vi "LIDAR V3 Mem2 Manager.vi"(11 "Source Name":refnum<k21>="100 MHz Clock") -> ()   [LabVIEW 2013]
uses:
  <vilib>/Platform/TimedLoop/XDataNode/wakeup.ctl
  <vilib>/Platform/TimedLoop/XDataNode/XDNodeRunTimeDep.lvlib
  <vilib>/Platform/TimedLoop/XDataNode/nitl_modes.ctl
  <vilib>/Platform/TimedLoop/XDataNode/timing_clust.ctl
  <vilib>/Platform/TimedLoop/XDataNode/XDataNode.xnode
  <vilib>/rvi/DataTransferAndStorage/Container/XNode/niFpgaContainer.xnode
  <vilib>/rvi/FXPMathLib/FxpAdd/XNode/nifxpmath_Add.xnode
  <vilib>/rvi/FXPMathLib/sim/FxpSim.dll
  <vilib>/rvi/LocalResourceManager/LocalResourceManager.xnode
  <vilib>/rvi/FIFO/Fifo_Resource/niFpgaFifoEmulationRefIn.vi
  <vilib>/rvi/FIFO/Fifo_Resource/nirvififoEmulationRead.vi
  <vilib>/rvi/FIFO/Fifo_Resource/nirvififoEmulationWrite.vi
  <vilib>/rvi/Memory/Memory_Emulation/nirvimemoryFastEmulation.vi
  <vilib>/rvi/Memory/Memory_Emulation/nirvimemoryEmulation.vi
  <vilib>/rvi/DataTransferAndStorage/Container/Common/niFpgaContainerGetUniqueNameForEmu.vi
  <vilib>/rvi/DataTransferAndStorage/Container/Common/niFpgaContainerSetEmuInfo.vi
  <vilib>/rvi/eio/common/nirviEmuReportErrorAndStop.vi
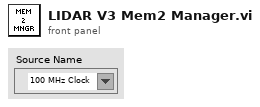
[diagram p1: front panel]
types:
  T1 = typedef "XDNodeRunTimeDep.lvlib/timing_clust.ctl" = cluster{"Expected End [f-1]":u64, "Actual End [f-1]":u64, "Finished Late? [f-1]":bool, "Expected End [i-1]":u64, "Actual End [i-1]":u64, "Finished Late? [i-1]":bool, "Expected Start [i]":u64, "Actual Start [i]":u64, "Expected Start [f]":u64, "Actual Start [f]":u64, "Source Name":string, "Structure Name":string, "Period":i64, "Deadline":i64, "Offset":i64, "Start":i64, "Priority":i32, "Timeout":i32, "Mode":T2, "Wakeup Reason":T3, "Error":errorcluster, "Source Type":string, "Secondary Source Type":string, "Global End Time":u64, "Global Start Time":u64, "Frame Duration":u64, "Iteration Duration":u64, "Assigned CPU":i32, "I/O Scan Engine Mode":u32}
  T2 = typedef "XDNodeRunTimeDep.lvlib/nitl_modes.ctl" = enum32{"No Change", "Process missed periods, maintain original phase", "Discard missed periods, maintain original phase", "Process missed periods, ignore original phase", "Discard missed periods, ignore original phase"}
  T3 = typedef "XDNodeRunTimeDep.lvlib/wakeup.ctl" = enum32{"Normal", "Aborted", "Asynchronous wakeup", "Timing source error", "Timed loop error", "Timeout"}
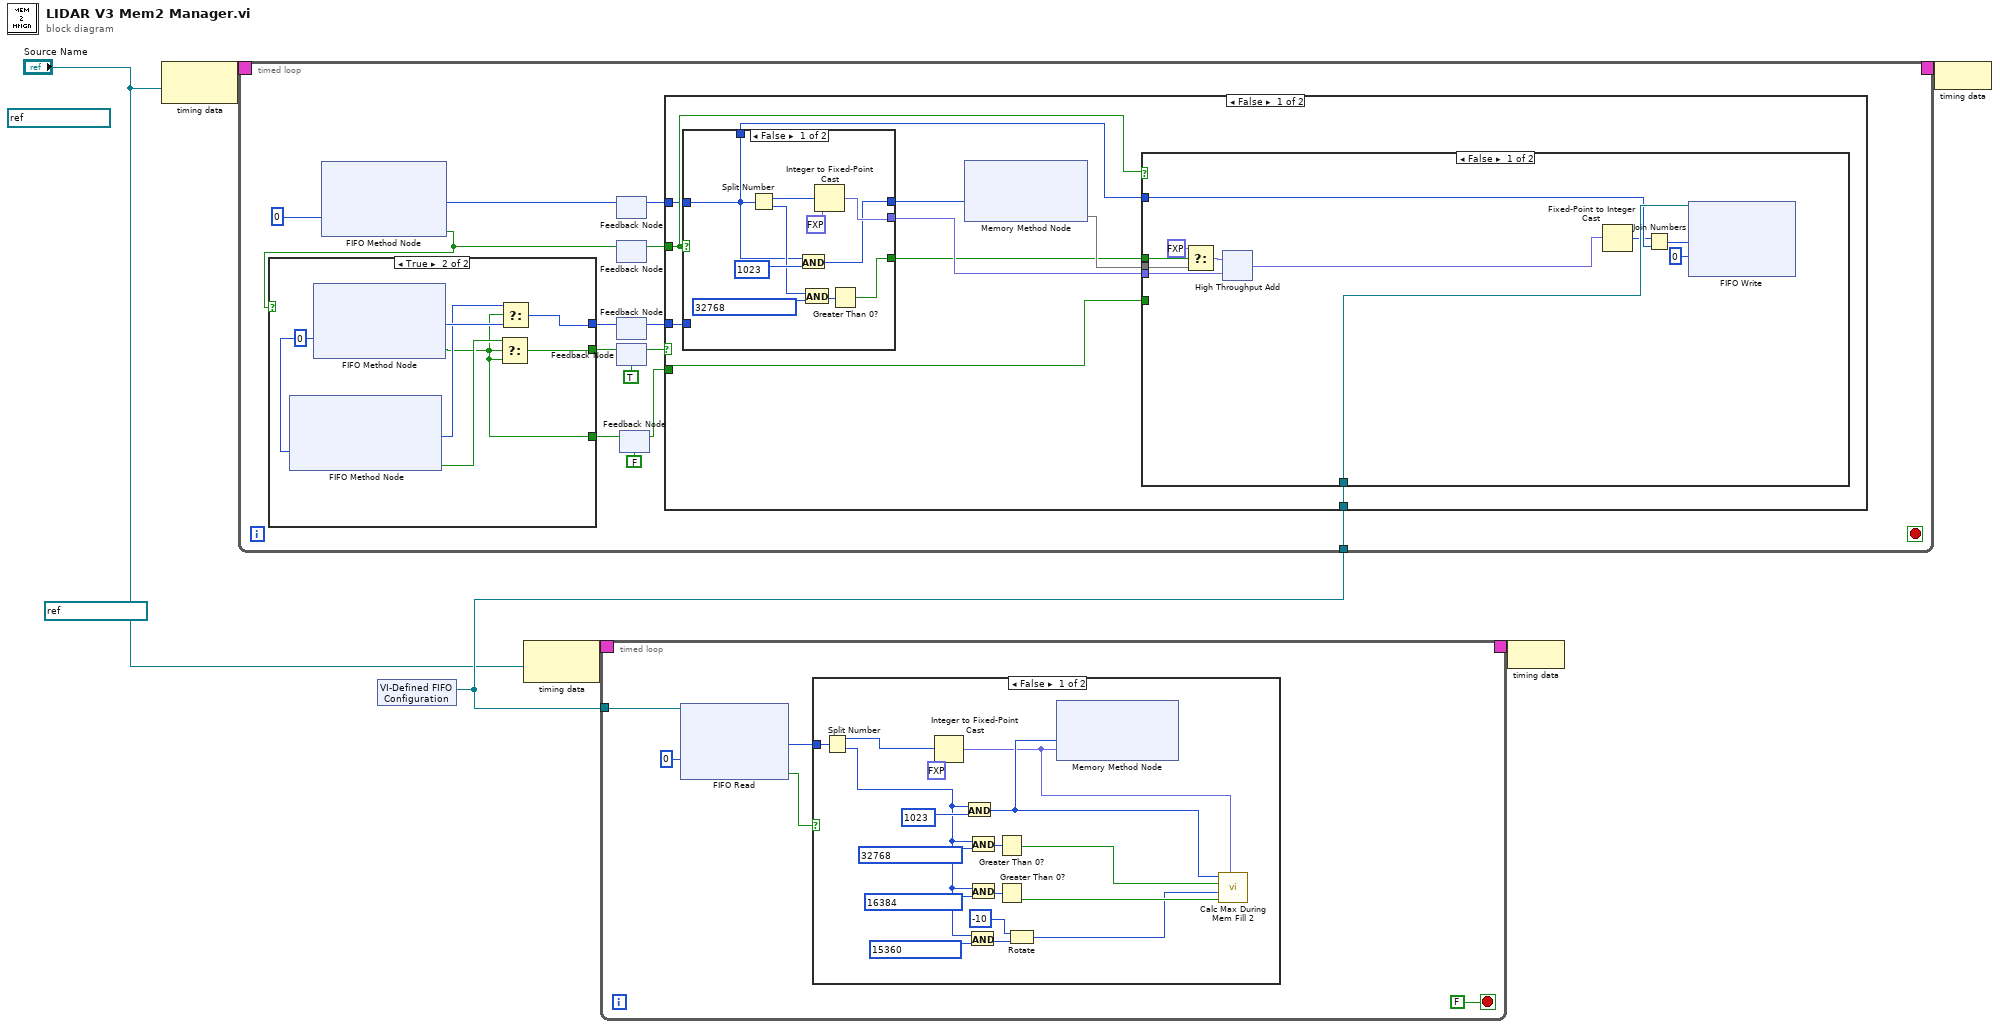
[diagram p0: block diagram]
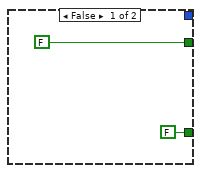
[diagram p3: hidden frame]
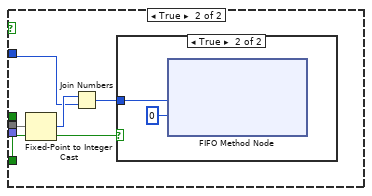
[diagram p4: hidden frame]
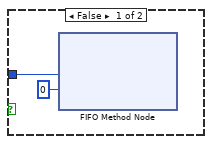
[diagram p5: hidden frame]
diagram:
  (unwired) refnum<k21> "100 MHz Clock" ("Source Name")
  (unwired) refnum<k21> "100 MHz Clock" ("Source Name")
  n1 = node-c288("Source Name") -> (w6:T1)
  n2 = xnode "VI-Defined FIFO Configuration"() -> ("FIFO Out"=w4:refnum<k21>)
  n3 = timed-loop {
    timing: w6 -> [_]
    timing-out: [_] -> w5
    tunnel: w4 -> [w15]
    stop <- _ stop-if-true
    n4 = xnode ("FIFO Method Node")("Timeout"=0) -> ("Element"=w20:u32, "Timed Out?"=w17:bool)  [unwired: 1 in, 1 out]
    n5 = case shown="True" w17 {
      tunnel: [FALSE ("Timed Out?") w28] -> w18
      tunnel: [_ w24] -> w16
      tunnel: [FALSE ("Timed Out?") w23] -> w9
      frame False {
      }
      frame True {
        w26 = 0 ("Timeout")
        n6 = xnode ("FIFO Method Node")("Timeout"=w26) -> ("Element"=w25:u32, "Timed Out?"=w29:bool)  [unwired: 1 in, 1 out]
        n7 = xnode ("FIFO Method Node")("Timeout"=w26) -> ("Element"=w27:u32, "Timed Out?"=w23:bool)  [unwired: 1 in, 1 out]
        n8 = Select(t=w29, s=w23, f=w23) -> (s? t:f=w28:bool)
        n9 = Select(t=w25, s=w23, f=w27) -> (s? t:f=w24:u32)
      }
    }
    n10 = feedback-in #1(w20) -> ()
    n11 = feedback #1() -> (w14:u32)  [unwired: 1 in]
    n12 = feedback-in #2(w17) -> ()
    n13 = feedback #2() -> (w13:bool)  [unwired: 1 in]
    n14 = feedback-in #3(w16) -> ()
    n15 = feedback #3() -> (w12:u32)  [unwired: 1 in]
    n16 = feedback-in #4(w18) -> ()
    n17 = feedback #4(TRUE ("Timed Out?")) -> (w11:bool)
    n18 = feedback #5(FALSE ("Timed Out?")) -> (w8:bool)
    n19 = feedback-in #5(w9) -> ()
    n20 = case shown="False" w11 {
      tunnel: w14 -> [w32 _]
      tunnel: w13 -> [w36 _]
      tunnel: w12 -> [w37 _]
      tunnel: w15 -> [w33 _]
      tunnel: w8 -> [w31 _]
      frame False {
        n21 = case shown="False" w36 {
          tunnel: w32 -> [w60 _]
          tunnel: [w69 _] -> w38
          tunnel: [w67 w70] -> w34
          tunnel: w37 -> [_ w70]
          tunnel: [w63 _] -> w35
          tunnel: [w60 w70] -> w30
          frame False {
            n22 = Split Number(x=w60) -> (hi(x)=w62:u16, lo(x)=w61:u16)
            n23 = And(x=w60, y=u32 1023) -> (x .and. y?=w67:u32)
            n24 = And(x=w61, y=u16 32768) -> (x .and. y?=w64:u16)
            n25 = Integer to Fixed-Point Cast(fixed-point type=fxp<+/-,16,16> 0.0, integer=w62) -> (fixed-point=w69:fxp<+/-,16,16>)
            n26 = Greater Than 0?(x=w64) -> (x > 0?=w63:bool)
          }
          frame True {
          }
        }
        n27 = xnode ("Memory Method Node")("Address"=w34) -> ("Data"=w39)  [unwired: 1 in, 1 out]
        n28 = case shown="False" w36 {
          tunnel: w39 -> [w48 w55]
          tunnel: w38 -> [w50 _]
          tunnel: w30 -> [w43 w52]
          tunnel: w35 -> [w44 _]
          tunnel: w33 -> [w45 _]
          tunnel: w31 -> [_ w51]
          frame False {
            n29 = Select(t=fxp<+/-,22,22> 0.0, s=w44, f=w48) -> (s? t:f=w47:fxp<+/-,22,22>)
            n30 = xnode ("High Throughput Add")("x"=w47, "y"=w50) -> ("x+y"=w46:fxp<+/-,22,22>)
            n31 = Fixed-Point to Integer Cast(1:w46) -> (0:w40:i32)
            n32 = Join Numbers(hi=w40, lo=w43) -> ((hi.lo)=w41:u64)
            n33 = xnode ("FIFO Write")("Element"=w41, "Timeout"=0, "FIFO In"=w45) -> ()  [unwired: 2 out]
          }
          frame True {
            n34 = Fixed-Point to Integer Cast(1:w55) -> (0:w53:i32)
            n35 = Join Numbers(hi=w53, lo=w52) -> ((hi.lo)=w54:u64)
            n36 = case shown="True" w51 {
              tunnel: w54 -> [w56 w58]
              frame False {
                n37 = xnode ("FIFO Method Node")("Element"=w56, "Timeout"=0) -> ()  [unwired: 1 in, 2 out]
              }
              frame True {
                n38 = xnode ("FIFO Method Node")("Element"=w58, "Timeout"=0) -> ()  [unwired: 1 in, 2 out]
              }
            }
          }
        }
      }
      frame True {
      }
    }
  }
  n39 = node-c288("Source Name") -> (w3:T1)
  n40 = timed-loop {
    tunnel: w4 -> [w75]
    timing: w3 -> [_]
    timing-out: [_] -> w2
    stop <- FALSE stop-if-true
    n41 = xnode ("FIFO Read")("Timeout"=0, "FIFO In"=w75) -> ("Element"=w77:u64, "Timed Out?"=w73:bool)  [unwired: 1 out]
    n42 = case shown="False" w73 {
      tunnel: w77 -> [w94 _]
      frame False {
        n43 = Split Number(x=w94) -> (hi(x)=w86:u32, lo(x)=w85:u32)
        n44 = Integer to Fixed-Point Cast(fixed-point type=fxp<+/-,22,22> 0.0, integer=w86) -> (fixed-point=w82:fxp<+/-,22,22>)
        n45 = And(x=w85, y=u32 1023) -> (x .and. y?=w83:u32)
        n46 = And(x=w85, y=u32 15360) -> (x .and. y?=w80:u32)
        n47 = And(x=w85, y=u32 32768) -> (x .and. y?=w90:u32)
        n48 = And(x=w85, y=u32 16384) -> (x .and. y?=w91:u32)
        n49 = Greater Than 0?(x=w90) -> (x > 0?=w84:bool)
        n50 = Greater Than 0?(x=w91) -> (x > 0?=w81:bool)
        n51 = Rotate(1:w80, 2:i8 -10 ("x")) -> (0:w79:u32)
        n52 = xnode ("Memory Method Node")("Address"=w83, "Data"=w82) -> ()  [unwired: 1 in, 1 out]
        n53 = call "Calc Max During Mem Fill 2.vi"("Value"=w82, "LastIterration"=w81, "ActiveLedIndex"=w79, "FirstIterration"=w84, "Address"=w83) -> ()  [unwired: 7 in]
      }
      frame True {
      }
    }
  }
  n54 = node-c288(w2) -> ()
  n55 = node-c288(w5) -> ()
